vi "读取队列输出.vi"(8 "error in (no error)":errorcluster caption="错误输入（无错误）", 11 "控制盒（队列）输入":refnum<class "控制盒（队列）.lvclass">) -> (0 "error out":errorcluster caption="错误输出", 2 "队列输出":refnum<queue>, 3 "控制盒（队列）输出":refnum<class "控制盒（队列）.lvclass">)   [LabVIEW 2011, in "控制盒（队列）.lvclass"]
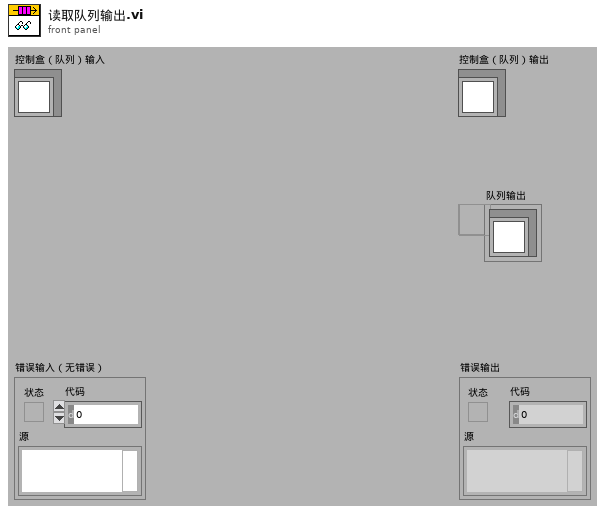
[diagram p1: front panel]
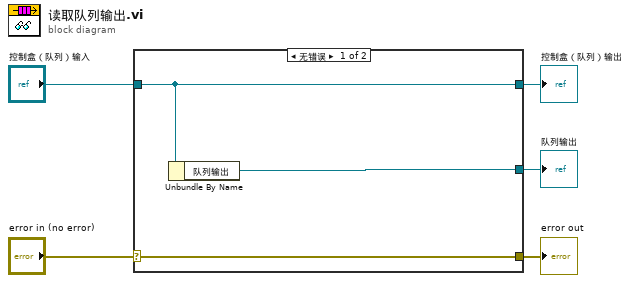
[diagram p0: block diagram]
diagram:
  n1 = case shown="无错误" "error in (no error)" {
    selector: "error in (no error)" -> [w8 w9]
    tunnel: [w8 w9] -> w4
    tunnel: [w7 w10] -> w2
    tunnel: "控制盒（队列）输入" -> [w7 w10]
    tunnel: [w6 _] -> w1
    frame No Error {
      n2 = Unbundle By Name(w7) -> ("队列输出"=w6:refnum<queue>)
    }
    frame Error {
    }
  }
  "error out" <- w4
  "控制盒（队列）输出" <- w2
  "队列输出" <- w1
